vi "FSM_Create.vi"(6 "initial state":string, 8 "error in (no error)":errorcluster, 9 "states":string[](array[string]), 10 "base path":path, 11 "FSM name":string) -> (0 "error out":errorcluster, 3 "FSM":refnum<class "FSM.lvclass">)   [LabVIEW 2021, in "FSM.lvclass"]
doc: "Create a Finite State Machine instance.\n\nCallback VIs should be created on base directory in order to be invoked lateer by FSM_Exec\n\nAuthor: J. Camilo Gomez C."
uses:
  FSM.lvclass
  FSM.lvclass/FSM.ctl
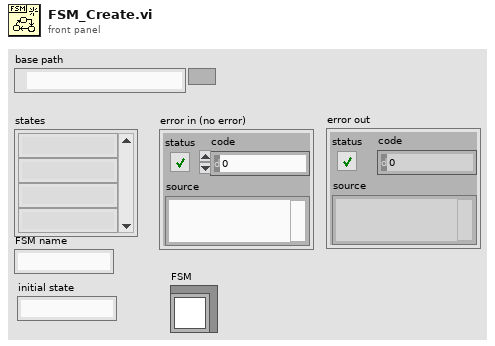
[diagram p1: front panel]
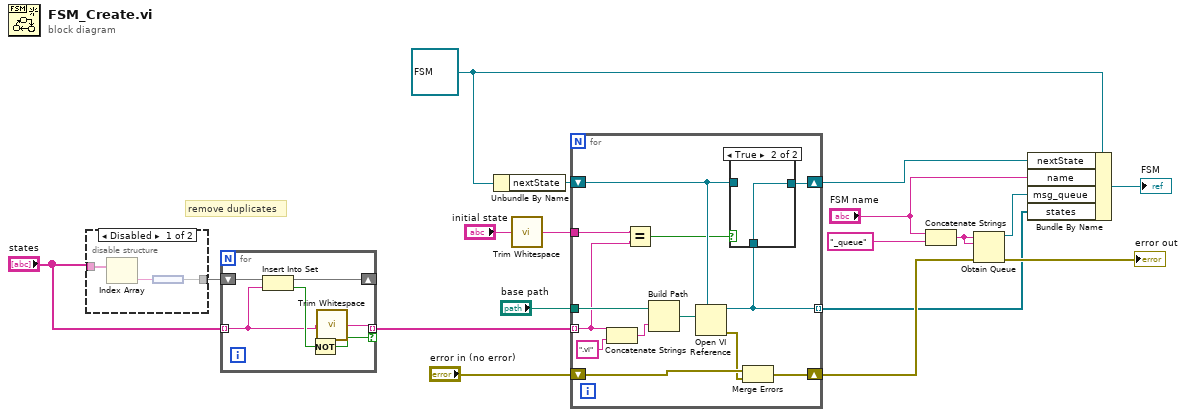
[diagram p0: block diagram]
diagram:
  w6 = refnum<class "FSM.lvclass"> refnum ("FSM.lvclass")
  # "remove duplicates"
  n1 = disable-structure shown="Disabled" {
    disable-tunnel: [w20 _] -> w9
    disable-tunnel: "states" -> [w19 _]
    frame Disabled {
      n2 = Index Array(array=w19) -> (element=w21:string)  [unwired: 1 in]
      n3 = node(w21) -> (w20:set{string})
    }
    frame Enabled {
    }
  }
  n4 = for {
    shift-right: [w26] -> _
    shift-left: w9 -> [w27]
    tunnel: "states" -> [w23] mode=indexing
    tunnel: [w22] -> w7 mode=indexing if=w24
    n5 = Insert Into Set(10:w23, 11:w27) -> (2:w25:bool, 3:w26:set{string})
    n6 = Not(x=w25) -> (.not. x?=w24:bool)
    n7 = call <vilib>:"Trim Whitespace.vi"("string"=w23) -> ("trimmed string"=w22:string)  [unwired: 1 in]
  }
  n8 = Unbundle By Name(w6) -> ("nextState"=w5:refnum<vi>)
  n9 = call <vilib>:"Trim Whitespace.vi"("string"="initial state") -> ("trimmed string"=w1:string)  [unwired: 1 in]
  n10 = for {
    tunnel: "base path" -> [w40]
    tunnel: w7 -> [w29] mode=indexing
    tunnel: [w32] -> w4 mode=indexing
    shift-right: [w36] -> w14
    shift-left: "error in (no error)" -> [w35]
    shift-right: [w33] -> w3
    shift-left: w5 -> [w31]
    tunnel: w1 -> [w30]
    n11 = Concatenate Strings(w29, ".vi" ("string")) -> (w38:string)
    n12 = Equal?(x=w30, y=w29) -> (x = y?=w28:bool)
    n13 = Build Path(base path=w40, name or relative path=w38) -> (appended path=w37:path)
    n14 = Open VI Reference(type specifier VI Refnum (for type only)=w31, vi path=w37) -> (vi reference=w32:refnum<vi>, error out=w34:errorcluster)  [unwired: 4 in]
    n15 = case shown="True" w28 {
      tunnel: w31 -> [w41 _]
      tunnel: [w41 w42] -> w33
      tunnel: w32 -> [_ w42]
      frame False {
      }
      frame True {
      }
    }
    n16 = Merge Errors(w35, w34) -> (w36:errorcluster)
  }
  n17 = Concatenate Strings("FSM name", "_queue" ("string")) -> (w16:string)
  n18 = Obtain Queue(name (unnamed)=w16, element data type=w16, error in (no error)=w14) -> (queue out=w11:refnum<queue>, error out=→"error out":errorcluster)  [unwired: 2 in, 1 out]
  n19 = Bundle By Name(cluster=w6, "nextState"=w3, "name"="FSM name", "msg_queue"=w11, "states"=w4) -> (→"FSM":refnum<class "FSM.lvclass">)
